vi "Sensor inout without fpga optimised.vi"(6 "Degrees":dbl, 8 "error in (no error)":errorcluster, 9 "sensor y":i32, 10 "Sensor x":i32, 11 "map reference in":refnum<data-value>) -> (0 "error out":errorcluster, 3 "map reference out 2":refnum<data-value>)   [LabVIEW 2012]
uses:
  <vilib>/robotics/Navigation/shared/WorldMap/OccupancyGridWorldMap/NI_Robotics_OccupancyGridWorldMap.lvclass
panel:
  out "Rounded y":fxp<+/-,64,32>
  out "Rounded x":fxp<+/-,64,32>
  out "Detected x":fxp<+/-,64,32>
  out "Detected y":fxp<+/-,64,32>
  in  "distance":dbl
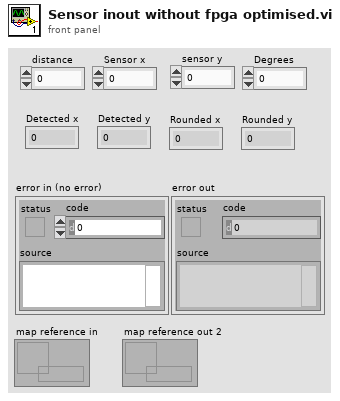
[diagram p1: front panel]
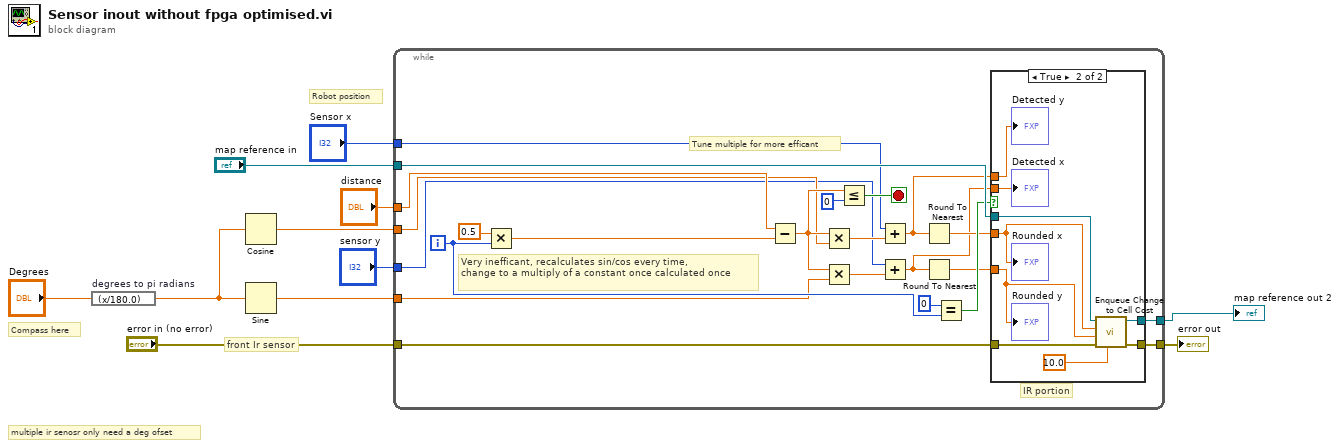
[diagram p0: block diagram]
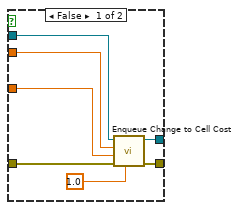
[diagram p2: hidden frame]
diagram:
  # "multiple ir senosr only need a deg ofset"
  # "Robot position"
  # "front Ir sensor"
  # "Compass here"
  n1 = expression code="(x/180.0)" "degrees to pi radians"("Degrees") -> (w3:dbl)
  n2 = Cosine(x=w3) -> (cos(x)=w1:dbl)
  n3 = Sine(x=w3) -> (sin(x)=w2:dbl)
  n4 = while {
    tunnel: "map reference in" -> [w34]
    tunnel: "error in (no error)" -> [w33]
    tunnel: [w32] -> w10
    tunnel: [w31] -> w11
    tunnel: "sensor y" -> [w13]
    tunnel: "Sensor x" -> [w12]
    tunnel: "distance" -> [w21]
    tunnel: w2 -> [w18]
    tunnel: w1 -> [w19]
    i -> [w26]
    stop <- w22 stop-if-true
    # "Tune multiple for more efficant"
    # "IR portion"
    # "Very inefficant, recalculates sin/cos every time, \nchange to a multiply of a constant once calculated once"
    n5 = Multiply(x=0.5, y=w26) -> (x*y=w24:dbl)
    n6 = Subtract(x=w21, y=w24) -> (x-y=w20:dbl)
    n7 = Multiply(x=w20, y=w19) -> (x*y=w17:dbl)
    n8 = Multiply(x=w20, y=w18) -> (x*y=w16:dbl)
    n9 = Less Or Equal?(x=w20, y=0) -> (x <= y?=w22:bool)
    n10 = Add(x=w12, y=w17) -> (x+y=w15:dbl)
    n11 = Add(x=w13, y=w16) -> (x+y=w14:dbl)
    n12 = Round To Nearest(number=w15) -> (nearest integer value=w27:dbl)
    n13 = Round To Nearest(number=w14) -> (nearest integer value=w28:dbl)
    n14 = Equal?(x=0, y=w26) -> (x = y?=w29:bool)
    n15 = case shown="True" w29 {
      tunnel: w34 -> [w37 w50]
      tunnel: w33 -> [w38 w49]
      tunnel: [w40 w47] -> w32
      tunnel: [w39 w46] -> w31
      tunnel: w27 -> [w36 w44]
      tunnel: w28 -> [w35 w45]
      tunnel: w15 -> [_ w43]
      tunnel: w14 -> [_ w42]
      frame False {
        n16 = call <vilib>:"Enqueue Change to Cell Cost.vi"("cost"=1.0, "error in (no error)"=w38, "y"=w35, "x"=w36, "map reference in"=w37) -> ("error out"=w39:errorcluster, "map reference out"=w40:refnum<data-value>)  [unwired: 5 in]
      }
      frame True {
        n17 = call <vilib>:"Enqueue Change to Cell Cost.vi"("cost"=10.0, "error in (no error)"=w49, "y"=w45, "x"=w44, "map reference in"=w50) -> ("error out"=w46:errorcluster, "map reference out"=w47:refnum<data-value>)  [unwired: 5 in]
        "Rounded y" <- w45
        "Rounded x" <- w44
        "Detected x" <- w42
        "Detected y" <- w43
      }
    }
  }
  "map reference out 2" <- w10
  "error out" <- w11
